vi "ITM10_Main.vi"() -> ()   [LabVIEW 2019]
doc: "Perform the acquisition. Replace the contents of this diagram with calls to acquisition hardware.\n_____\nBased on Delacor QMH Project Template 5.0.0.82."
uses:
  ITM10_Global.vi
panel:
  out "temperature":dbl[](array[numeric]) format="%.1f"
  out "status_log":bool caption="Status"
  out "Last Measurement":timestamp format="%<%Y-%m-%d %H:%M:%S>T"
  in  "stop":bool
  in  "Logging":bool=TRUE
  out "Chart":waveform(dbl)[](graph)
  out "Status":bool
  in  "Interval":dbl=5.0 caption="sec" format="%#_13g"
  in  "VISA":refnum<visa-resource-name>="COM34"
  # "Oxford ITM10 :  Magnet Coil Temperature"
  # "Chart-Axis Control"
  # "Ch 1: Tank T"
  # "K"
  # "Ch 2: Tank B"
  # "K"
  # "K"
  # "Ch 3: Coil T"
  # "Ch 4: Coil B"
  # "K"
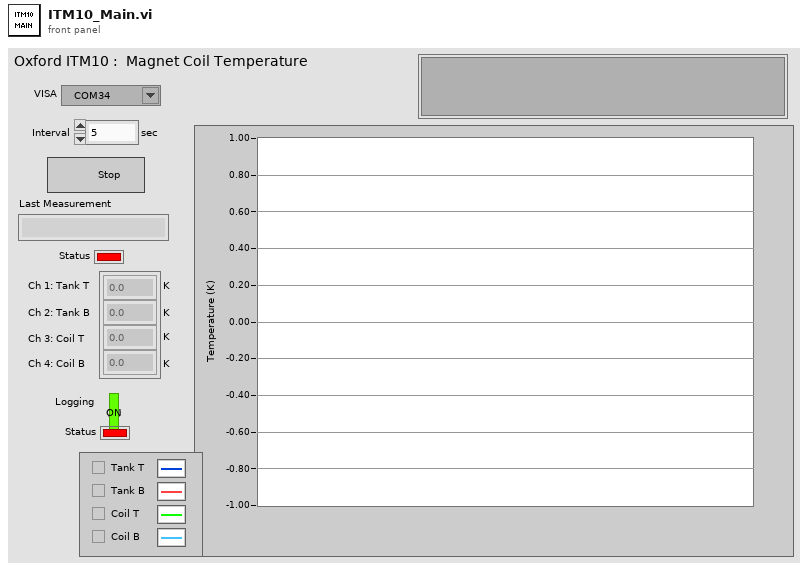
[diagram p1: front panel]
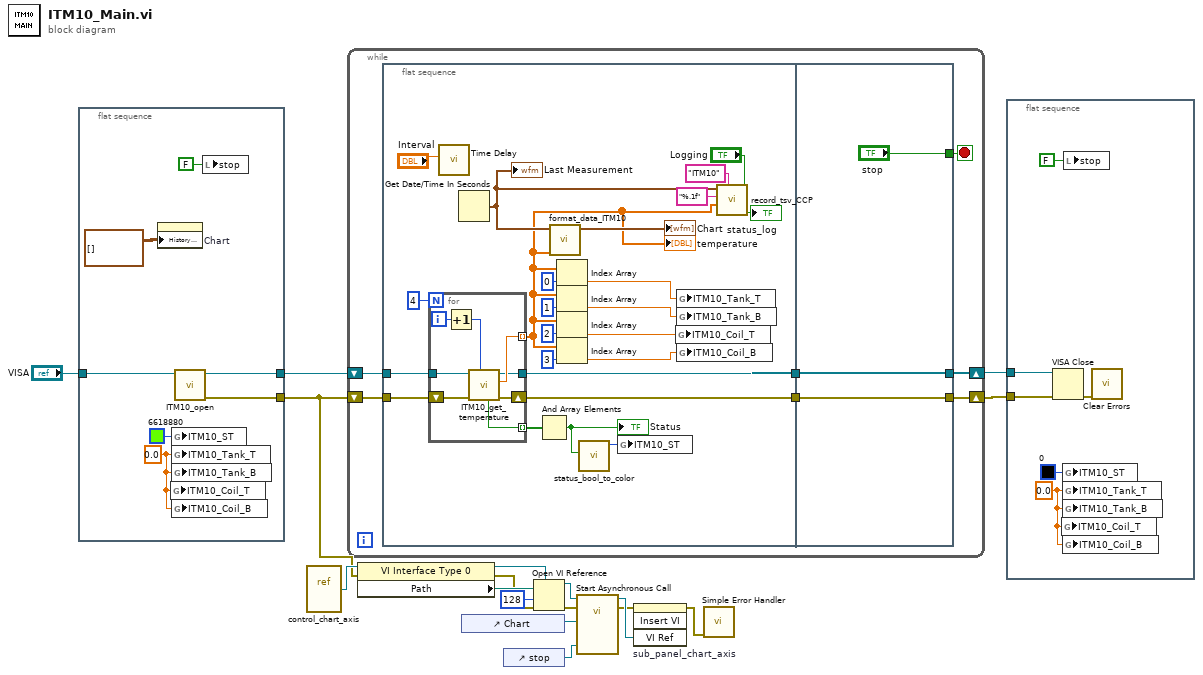
[diagram p0: block diagram]
diagram:
  n1 = flat-sequence {
    tunnel: [w20] -> w5
    tunnel: [w21] -> w15
    tunnel: "VISA" -> [w22]
    frame #0 {
      w19 = 0.0 ("ITM10_Tank_T")
      n2 = property on="Chart" class="WFChart (strict)"("History Data"=waveform(dbl)[][] []) -> ()  [unwired: 2 in, 2 out]
      n3 = global write "ITM10_Global.vi" "ITM10_Coil_T"(w19) -> ()
      n4 = global write "ITM10_Global.vi" "ITM10_ST"(u32 6618880 ("ITM10_ST")) -> ()
      n5 = global write "ITM10_Global.vi" "ITM10_Tank_T"(w19) -> ()
      n6 = global write "ITM10_Global.vi" "ITM10_Tank_B"(w19) -> ()
      n7 = global write "ITM10_Global.vi" "ITM10_Coil_B"(w19) -> ()
      n8 = call "ITM10_open.vi"("VISA in"=w22) -> ("error out"=w20:errorcluster, "VISA out"=w21:refnum<visa-resource-name>)  [unwired: 9 in]
      n9 = local write "stop"(FALSE ("stop")) -> ()
    }
  }
  n10 = vi-ref "control_chart_axis.vi"() -> (w10:refnum<vi>)
  n11 = while {
    shift-right: [w29] -> w17
    shift-left: w15 -> [w31]
    shift-right: [w28] -> w16
    shift-left: w5 -> [w30]
    stop <- w25 stop-if-true
    n12 = flat-sequence {
      tunnel: w31 -> [w48]
      tunnel: w30 -> [w49]
      tunnel: [w46] -> w27
      tunnel: [w47] -> w26
      tunnel: [w65] -> w28
      tunnel: [w66] -> w29
      tunnel: w27 -> [w66]
      tunnel: w26 -> [w65]
      tunnel: ["stop"] -> w25
      frame #0 {
        n13 = for {
          N: 4 -> [_]
          tunnel: w48 -> [w62]
          tunnel: [w60] -> w36 mode=indexing
          tunnel: [w59] -> w46
          tunnel: [w58] -> w45 mode=indexing
          shift-right: [w61] -> w47
          shift-left: w49 -> [w63]
          i -> [w57]
          n14 = Increment(x=w57) -> (x+1=w56:i32)
          n15 = call "ITM10_get_temperature.vi"("channel"=w56, "err_in"=w63, "visa_in"=w62) -> ("err_out"=w61:errorcluster, "temp"=w60:dbl, "visa_out"=w59:refnum<visa-resource-name>, "status"=w58:bool)  [unwired: 4 in, 1 out]
        }
        "temperature" <- w36
        n16 = call "Time Delay"("Delay Time (s)"="Interval") -> ()  [unwired: 10 in, 1 out]
        n17 = Get Date/Time In Seconds() -> (seconds since 1Jan1904=w51:timestamp)
        "Last Measurement" <- w51
        n18 = And Array Elements(Boolean array=w45) -> (logical AND=w42:bool)
        "Status" <- w42
        n19 = call "format_data_ITM10.vi"("value_array"=w36, "time"=w51) -> ("waveform_array"=→"Chart":waveform(dbl)[])  [unwired: 9 in]
        n20 = Index Array(array=w36, index=0) -> (element=w35:dbl)
        n21 = Index Array(array=w36, index=1) -> (element=w34:dbl)
        n22 = Index Array(array=w36, index=2) -> (element=w33:dbl)
        n23 = Index Array(array=w36, index=3) -> (element=w32:dbl)
        n24 = call "status_bool_to_color.vi"("status_bool_2"=w42) -> ("status_color"=w41:u32)  [unwired: 10 in]
        n25 = global write "ITM10_Global.vi" "ITM10_ST"(w41) -> ()
        n26 = global write "ITM10_Global.vi" "ITM10_Coil_T"(w33) -> ()
        n27 = global write "ITM10_Global.vi" "ITM10_Tank_T"(w35) -> ()
        n28 = global write "ITM10_Global.vi" "ITM10_Tank_B"(w34) -> ()
        n29 = global write "ITM10_Global.vi" "ITM10_Coil_B"(w32) -> ()
        n30 = call "record_tsv_CCP.vi"("logging_on"="Logging", "folder_name"="ITM10", "value_array"=w36, "format"="%.1f", "time"=w51) -> ("status"=→"status_log":bool)  [unwired: 5 in, 1 out]
      }
      frame #1 {
      }
    }
  }
  n31 = property class="VI Interface Type 0"(reference=w10, error in=w5) -> (reference out=w7:refnum<vi>, error out=w4:errorcluster, "Path"=w11:path)
  n32 = control-ref of="Chart"() -> (w6:refnum<vi>)
  n33 = control-ref of="stop"() -> (w13:refnum<vi>)
  n34 = Open VI Reference(type specifier VI Refnum (for type only)=w7, vi path=w11, options=128, error in (no error)=w4) -> (vi reference=w9:refnum<vi>, error out=w3:errorcluster)  [unwired: 2 in]
  n35 = call-by-ref "Start Asynchronous Call"(reference=w9, error in=w3, "stop"=w13, "chart_1"=w6) -> (reference out=w12:refnum<vi>, error out=w2:errorcluster)  [unwired: 10 in]
  n36 = invoke on="sub_panel_chart_axis" class="SubPnl" method="Insert VI"(error in=w2, "VI Ref"=w12) -> (error out=w1:errorcluster)  [unwired: 2 in, 3 out]
  n37 = call <vilib>:"Simple Error Handler.vi"("error in (no error)"=w1) -> ()  [unwired: 4 in, 5 out]
  n38 = flat-sequence {
    tunnel: w17 -> [w72]
    tunnel: w16 -> [w71]
    frame #0 {
      w68 = 0.0 ("ITM10_Tank_T")
      n39 = VISA Close(VISA resource name=w72, error in (no error)=w71) -> (error out=w70:errorcluster)
      n40 = global write "ITM10_Global.vi" "ITM10_Coil_T"(w68) -> ()
      n41 = global write "ITM10_Global.vi" "ITM10_ST"(u32 0 ("ITM10_ST")) -> ()
      n42 = global write "ITM10_Global.vi" "ITM10_Tank_T"(w68) -> ()
      n43 = global write "ITM10_Global.vi" "ITM10_Tank_B"(w68) -> ()
      n44 = global write "ITM10_Global.vi" "ITM10_Coil_B"(w68) -> ()
      n45 = local write "stop"(FALSE ("stop")) -> ()
      n46 = call <vilib>:"Clear Errors.vi"("error in (no error)"=w70) -> ()  [unwired: 5 in, 2 out]
    }
  }
